vi "Calculate Baseline.vi"(6 "baselineThreshold":u16, 8 "traceLength":i32, 9 "data_12_bit":u16[](array[numeric]), 10 "baselineLength":i32, 11 "error in (no error)":errorcluster) -> (0 "Stdev":i16, 1 "Baseline":i16, 3 "error out":errorcluster)   [LabVIEW 2013]
doc: "<B>Explanation of params</B>\nA description is included at the bottom.\n<B>int32_t errorValue</B>: The return value for the function, a 0 (zero) means a baseline is found,\n a value >= 5000 indicates the occurrence of an error.\n<B>int32_t defaultStart</B>: The initial starting value for calculating the baseline, in most cases \n this value should be 0 (zero). This value can only be adjusted in this VI and has\n no external control.\n<B>int32_t baselineLength</B>: The initial - this can change because the function is recursive and \n hence can update this value - maximum element that is included in the baseline.\n If a pulse occurres before this element the calculation stops there.\n<B>uint16_t data_12_bit[]</B>: The array which holds the event data.\n<B>const int32_t traceLength</B>: The size of the event data array.\n<B>const uint16_t baselineThreshold</B>: This value determines if an element is part of the baseline or\n belongs to a pulse. The threshold works on both sides of the baseline i.e. both the \n positive and the negative.\n<B>const int32_t minimalInBaseline</B>: Defines the minimal number of elements that should be\n present in the baseline. This value is by default wired to <B>baselineLength</B>\n so that the length of the baselline is also the minimal number of elements in the\n trace. This is a separate parameter because the <B>baselineLength</B> as said\n before can be internally updated when running the VI. This value can only be\n adjusted in this VI and has no external control.\n <B>int16_t *Baseline</B>: A pointer to the calculated baseline. LABVIEW handles this as a\n pointer to value, so this value holds the baseline.\n<B>int16_t *Stdev</B>: A pointer to the calculated standard deviation. LABVIEW handles this as a\n pointer to value, so this value holds the standard deviation.\n\n<B>Description</B> \nThis Vi finds the baseline and corresponding standard deviation, providing an event data array with a supplied size. The initial baseline is calculated from <B>defaultStart</B> to <B>baselineLength</B>, by using the <B>baselineThreshold</B> to determine when an element is no longer part of the baseline. If the calculation stops before <B>minimalInBaseline</B> is reached, internally the new <B>defaultStart</B> is determined using two sequences i.e. subarrays of width 100 - defined in the DLL <B>sequence.h</B> header file Both sequences are compared and if the next sequence is less smooth than the current sequence the start of the current sequence is picked as the new starting point for calculating the baseline. In the end the baseline and standard deviation are returned. If no baseline can be found both the <B>Baseline</B> and the <B>Stdev</B> get a value of <B>-999</B>\n\n<B>Comply with the old implementation</B>\nIt is possible to mimic the old implementation by wiring the size of the array to <B>baselineLength</B> - so it determines the baseline until it hits a pulse, set the <B>minimalInBaseline</B> to 50 and the threshold to 25"
uses:
  <userlib>/Baseline/Baseline.lvlib
  project/Baseline/Release/Baseline.dll
panel:
  out "errorValue":i32
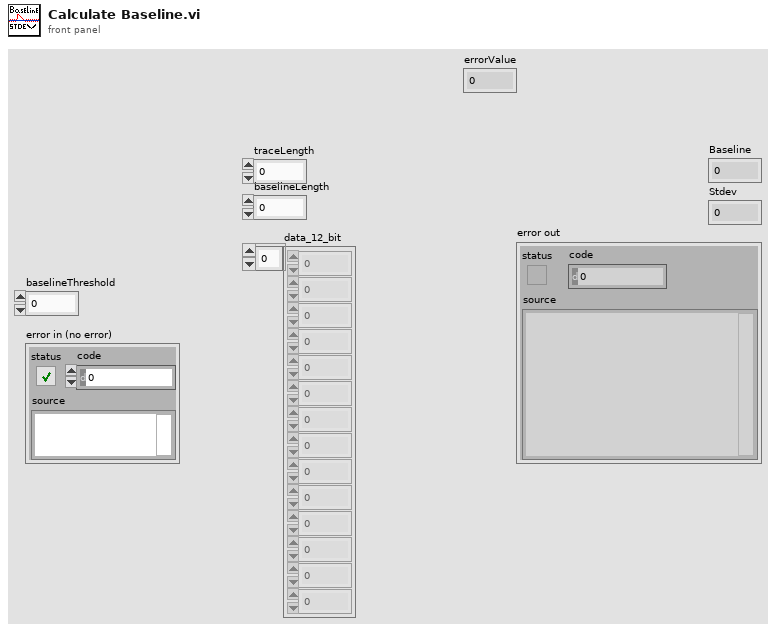
[diagram p1: front panel]
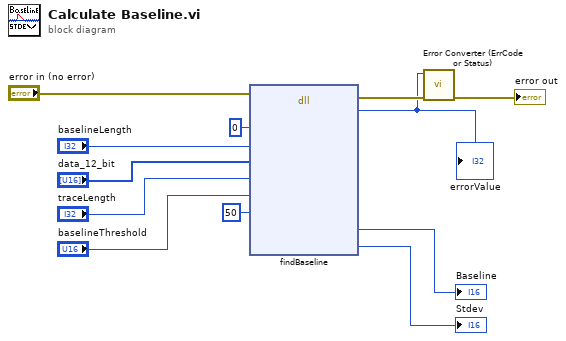
[diagram p0: block diagram]
diagram:
  n1 = dll-call lib="C:/Users/SuperUser/Documents/HiSparc/HISPARC_baseline/project/Baseline/Release/Baseline.dll" fn="findBaseline"(error in="error in (no error)", "defaultStart"=0, "baselineLength"="baselineLength", "data_12_bit"="data_12_bit", "traceLength"="traceLength", "baselineThreshold"="baselineThreshold", "minimalInBaseline"=50) -> (error out=w9:errorcluster, "errorValue"=w8:i32, "Baseline"=→"Baseline":i16, "Stdev"=→"Stdev":i16)  [unwired: 10 in, 1 out]
  "errorValue" <- w8
  n2 = call "Error Converter (ErrCode or Status).vi"("error in (no error)"=w9, "error code"=w8) -> ("error out"=→"error out":errorcluster)  [unwired: 9 in]
